vi "String to Flow Control.vi"(10 "Interface Type in":T1, 11 "value":string) -> (3 "Interface Type out":T1)   [LabVIEW 2015, in "Modbus Master System Explorer.lvlib"]
uses:
  Modbus Master System Explorer.lvlib
  Shared/Controls/Interface Type.ctl
  Shared/Modbus Master Shared.lvlib
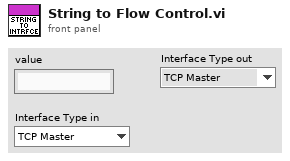
[diagram p1: front panel]
types:
  T1 = typedef "Modbus Master Shared.lvlib/Interface Type.ctl" = enum16{"TCP Master", "Serial Master"}
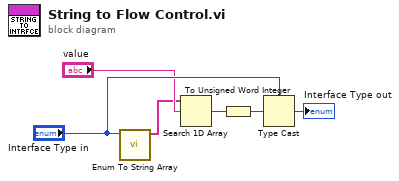
[diagram p0: block diagram]
diagram:
  n1 = call "Enum To String Array.vi"("Interface Type"="Interface Type in") -> ("Strings"=w1:string[])  [unwired: 10 in]
  n2 = Search 1D Array(1D array=w1, element="value") -> (index of element=w3:i32)  [unwired: 1 in]
  n3 = To Unsigned Word Integer(number=w3) -> (unsigned 16bit integer=w4:u16)
  n4 = Type Cast(type="Interface Type in", x=w4) -> (*(type *) &x=→"Interface Type out":T1)
